vi "CopyDefaultFile.vi"(6 "OriginFile":string, 8 "error in (no error)":errorcluster, 9 "DestFile":string, 10 "Origin":path, 11 "Destination":path) -> (0 "error out":errorcluster)   [LabVIEW 2014, in "Config_class.lvlib" / "Config.lvclass"]
uses:
  Config.lvclass
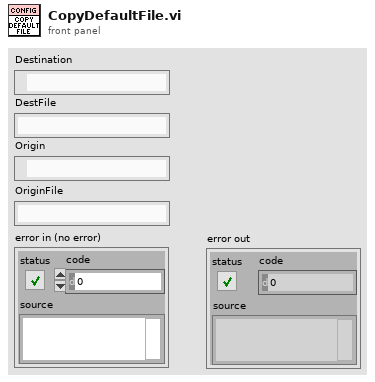
[diagram p1: front panel]
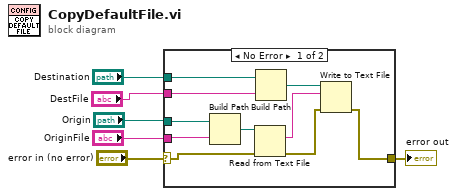
[diagram p0: block diagram]
diagram:
  n1 = case shown="No Error" "error in (no error)" {
    selector: "error in (no error)" -> [w10 w17]
    tunnel: [w9 w17] -> w5
    tunnel: "OriginFile" -> [w14 _]
    tunnel: "Destination" -> [w15 _]
    tunnel: "Origin" -> [w8 _]
    tunnel: "DestFile" -> [w7 _]
    frame No Error {
      n2 = Build Path(base path=w8, name or relative path=w14) -> (appended path=w16:path)
      n3 = Read from Text File(file (use dialog)=w16, error in=w10) -> (text=w12:string, error out=w11:errorcluster)  [unwired: 2 in, 2 out]
      n4 = Build Path(base path=w15, name or relative path=w7) -> (appended path=w13:path)
      n5 = Write to Text File(file (use dialog)=w13, text=w12, error in=w11) -> (error out=w9:errorcluster)  [unwired: 1 in, 2 out]
    }
    frame Error {
    }
  }
  "error out" <- w5
